vi "String To Value with no SI Prefix.vi"(8 "error in":errorcluster, 11 "Response":string) -> (0 "error out":errorcluster, 2 "Unit":T1, 3 "Scaled Value":dbl format="%#.6f")   [LabVIEW 2013, in "Mercury iXX.lvlib"]
uses:
  Mercury iXX.lvlib
  Controls/Unit String.ctl
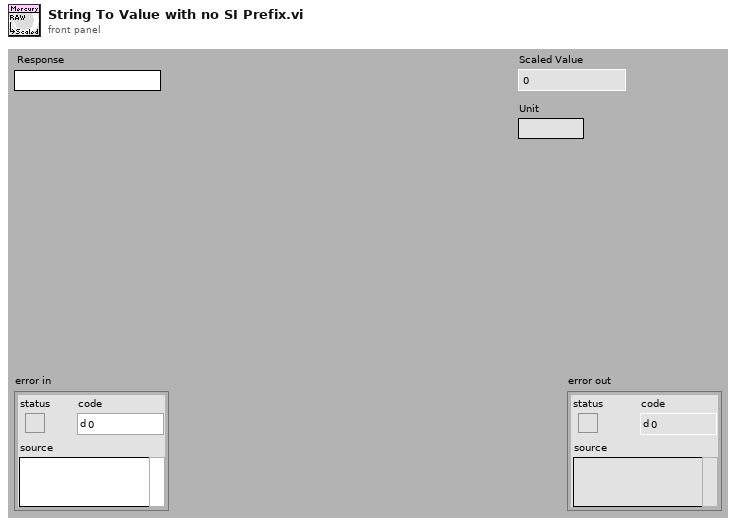
[diagram p1: front panel]
types:
  T1 = typedef "Mercury iXX.lvlib/Unit String.ctl" = string
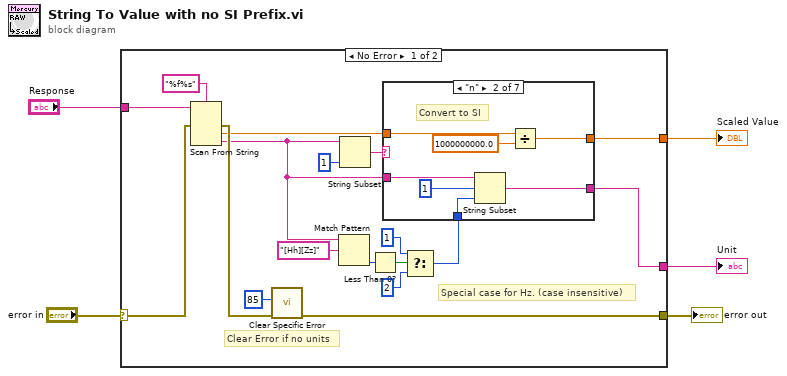
[diagram p0: block diagram]
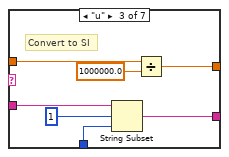
[diagram p3: hidden frame]
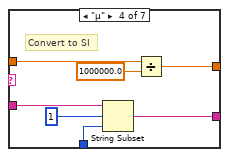
[diagram p4: hidden frame]
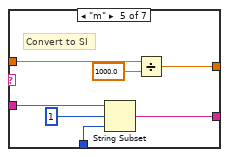
[diagram p5: hidden frame]
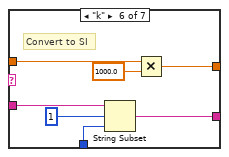
[diagram p6: hidden frame]
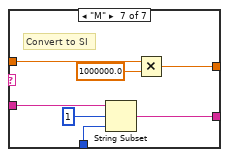
[diagram p7: hidden frame]
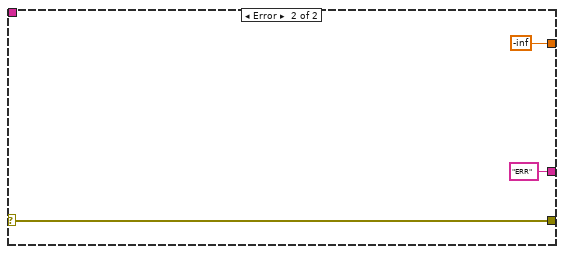
[diagram p8: hidden frame]
diagram:
  n1 = case shown="No Error" "error in" {
    selector: "error in" -> [w21 w70]
    tunnel: [w19 w70] -> w4
    tunnel: "Response" -> [w23 _]
    tunnel: [w7 -inf] -> w2
    tunnel: [w6 "ERR" ("Unit-")] -> w1
    frame No Error {
      # "Special case for Hz. (case insensitive)"
      # "Clear Error if no units"
      n2 = Scan From String(format string="%f%s", input string=w23, error in=w21) -> (error out=w20:errorcluster, output 1=w9:dbl, output 2=w8:string)  [unwired: 1 in, 4 out]
      n3 = call "Clear Specific Error.vi"("error in"=w20, "Code (-1:All)"=85) -> ("error out"=w19:errorcluster)  [unwired: 9 out]
      n4 = Match Pattern(string=w8, regular expression="[Hh][Zz]") -> (offset past match=w14:i32)  [unwired: 4 out]
      n5 = String Subset(string=w8, length (rest)=1 ("length (rest)")) -> (substring=w16:string)  [unwired: 1 out]
      n6 = Less Than 0?(x=w14) -> (x < 0?=w13:bool)
      n7 = Select(t=1 ("length (rest)"), s=w13, f=2) -> (s? t:f=w11:i32)
      n8 = case shown="\"n\"" w16 {
        tunnel: w9 -> [w25 w32 w39 w46 w53 w60 w67]
        tunnel: [w25 w30 w37 w44 w51 w58 w65] -> w7
        tunnel: w8 -> [w24 w29 w36 w43 w50 w57 w64]
        tunnel: [w24 w27 w34 w41 w48 w55 w62] -> w6
        tunnel: w11 -> [_ w26 w33 w40 w47 w54 w61]
        frame "", Default {
          # "Pass through SI units"
        }
        frame "n" {
          # "Convert to SI"
          n9 = String Subset(string=w29, offset (0)=1 ("length (rest)"), length (rest)=w26) -> (substring=w27:string)
          n10 = Divide(x=w32, y=1000000000.0) -> (x/y=w30:dbl)
        }
        frame "u" {
          # "Convert to SI"
          n11 = String Subset(string=w36, offset (0)=1 ("length (rest)"), length (rest)=w33) -> (substring=w34:string)
          n12 = Divide(x=w39, y=1000000.0) -> (x/y=w37:dbl)
        }
        frame "µ" {
          # "Convert to SI"
          n13 = String Subset(string=w43, offset (0)=1 ("length (rest)"), length (rest)=w40) -> (substring=w41:string)
          n14 = Divide(x=w46, y=1000000.0) -> (x/y=w44:dbl)
        }
        frame "m" {
          # "Convert to SI"
          n15 = String Subset(string=w50, offset (0)=1 ("length (rest)"), length (rest)=w47) -> (substring=w48:string)
          n16 = Divide(x=w53, y=1000.0) -> (x/y=w51:dbl)
        }
        frame "k" {
          # "Convert to SI"
          n17 = String Subset(string=w57, offset (0)=1 ("length (rest)"), length (rest)=w54) -> (substring=w55:string)
          n18 = Multiply(x=w60, y=1000.0) -> (x*y=w58:dbl)
        }
        frame "M" {
          # "Convert to SI"
          n19 = String Subset(string=w64, offset (0)=1 ("length (rest)"), length (rest)=w61) -> (substring=w62:string)
          n20 = Multiply(x=w67, y=1000000.0) -> (x*y=w65:dbl)
        }
      }
    }
    frame Error {
    }
  }
  "error out" <- w4
  "Scaled Value" <- w2
  "Unit" <- w1
